vi "Json Validate.vi"(6 "GenError(T)":bool=TRUE, 8 "error in (no error)":errorcluster, 11 "String":string) -> (0 "error out":errorcluster, 2 "Valid Json?":bool, 3 "Json without comments":string, 5 "String (dup)":string)   [LabVIEW 2019, in "lv-apt-json-file.lvlib"]
uses:
  lv-apt-json-file.lvlib
  <userlib>/NEVSTOP-Programming-Palette/Configuration/Ini/TextToLines.vi
  <userlib>/NEVSTOP-Programming-Palette/Configuration/Ini/LinesToText.vi
  <vilib>/Utility/error.llb/Error Cluster From Error Code.vi
  <vilib>/ErrorRing/Error Ring.xnode
  <vilib>/addons/_JKI.lib/Serialization/JSON/JKI JSON Serialization.lvlib
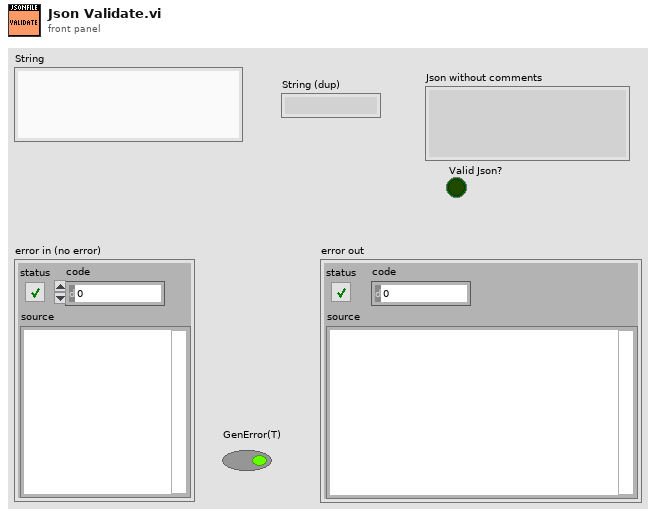
[diagram p1: front panel]
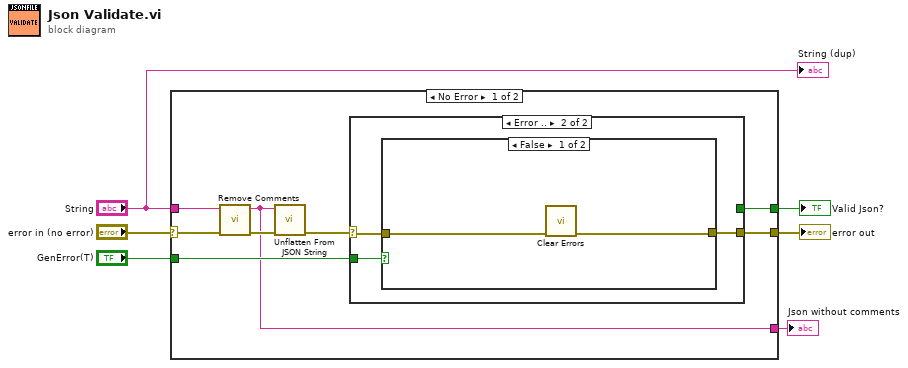
[diagram p0: block diagram]
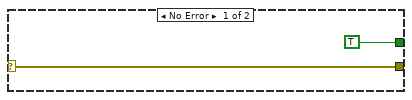
[diagram p2: hidden frame]
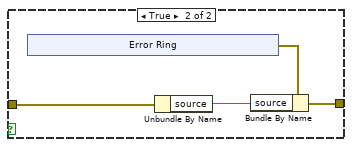
[diagram p3: hidden frame]
diagram:
  n1 = case shown="No Error" "error in (no error)" {
    selector: "error in (no error)" -> [w9 w30]
    tunnel: "String" -> [w10 _]
    tunnel: [w13 _] -> w5
    tunnel: [w12 w30] -> w4
    tunnel: "GenError(T)" -> [w11 _]
    tunnel: [w7 _] -> w1
    frame No Error {
      n2 = call "Remove Comments.vi"("error in (no error)"=w9, "String"=w10) -> ("error out"=w8:errorcluster, "string"=w7:string)  [unwired: 8 in]
      n3 = call <vilib>:"Unflatten From JSON String.vi"("error in (no error)"=w8, "JSON String"=w7) -> ("error out"=w14:errorcluster)  [unwired: 8 in, 1 out]
      n4 = case shown="Error .." w14 {
        selector: w14 -> [w15 w18]
        tunnel: [TRUE _] -> w13
        tunnel: [w15 w19] -> w12
        tunnel: w11 -> [_ w17]
        frame No Error {
        }
        frame Error {
          n5 = case shown="False" w17 {
            tunnel: [w20 w24] -> w19
            tunnel: w18 -> [w21 w23]
            frame False {
              n6 = call <vilib>:"Clear Errors.vi"("error in (no error)"=w21) -> ("error out"=w20:errorcluster)  [unwired: 5 in, 1 out]
            }
            frame True {
              n7 = xnode "Error Ring"() -> ("error out"=w25:errorcluster)
              n8 = Unbundle By Name(w23) -> ("source"=w22:string)
              n9 = Bundle By Name(cluster=w25, "source"=w22) -> (w24:errorcluster)
            }
          }
        }
      }
    }
    frame Error {
    }
  }
  "error out" <- w4
  "Valid Json?" <- w5
  "Json without comments" <- w1
  "String (dup)" <- "String"
